vi "Find Run.vi"(0 "Array":dbl[](array[numeric]), 5 "Condition":bool[](array[boolean]), 9 "Midrun index":i32) -> (4 "Run":dbl[](array[numeric]), 6 "Run start index":i32, 8 "Run end index":i32, 10 "Run length":i32)   [LabVIEW 2020]
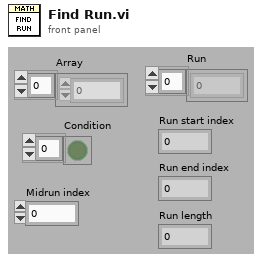
[diagram p1: front panel]
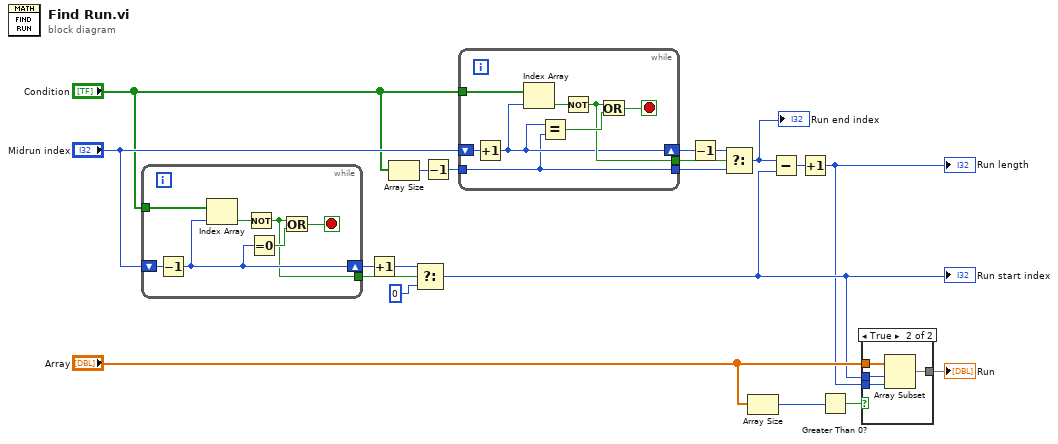
[diagram p0: block diagram]
diagram:
  n1 = while {
    shift-right: [w22] -> w19
    shift-left: "Midrun index" -> [w24]
    tunnel: "Condition" -> [w27]
    tunnel: [w21] -> w20
    stop <- w26 stop-if-true
    n2 = Decrement(x=w24) -> (x-1=w22:i32)
    n3 = Index Array(array=w27, index=w22) -> (element=w25:bool)
    n4 = Not(x=w25) -> (.not. x?=w21:bool)
    n5 = Equal To 0?(x=w22) -> (x = 0?=w23:bool)
    n6 = Or(x=w21, y=w23) -> (x .or. y?=w26:bool)
  }
  n7 = Increment(x=w19) -> (x+1=w18:i32)
  n8 = Array Size(array="Condition") -> (size(s)=w14:i32)
  n9 = Select(t=w18, s=w20, f=0) -> (s? t:f=w2:i32)
  "Run start index" <- w2
  n10 = Decrement(x=w14) -> (x-1=w13:i32)
  n11 = while {
    shift-right: [w29] -> w10
    shift-left: "Midrun index" -> [w32]
    tunnel: "Condition" -> [w35]
    tunnel: [w30] -> w11
    tunnel: w13 -> [w28]
    tunnel: [w28] -> w9
    stop <- w34 stop-if-true
    n12 = Increment(x=w32) -> (x+1=w29:i32)
    n13 = Index Array(array=w35, index=w29) -> (element=w33:bool)
    n14 = Equal?(x=w29, y=w28) -> (x = y?=w31:bool)
    n15 = Not(x=w33) -> (.not. x?=w30:bool)
    n16 = Or(x=w30, y=w31) -> (x .or. y?=w34:bool)
  }
  n17 = Decrement(x=w10) -> (x-1=w12:i32)
  n18 = Select(t=w12, s=w11, f=w9) -> (s? t:f=w8:i32)
  "Run end index" <- w8
  n19 = Array Size(array="Array") -> (size(s)=w3:i32)
  n20 = Subtract(x=w8, y=w2) -> (x-y=w7:i32)
  n21 = Increment(x=w7) -> (x+1=w1:i32)
  "Run length" <- w1
  n22 = Greater Than 0?(x=w3) -> (x > 0?=w4:bool)
  n23 = case shown="True" w4 {
    tunnel: "Array" -> [_ w39]
    tunnel: [_ w38] -> w6
    tunnel: w2 -> [_ w37]
    tunnel: w1 -> [_ w36]
    frame False {
    }
    frame True {
      n24 = Array Subset(array=w39, index=w37, length=w36) -> (w38:dbl[])
    }
  }
  "Run" <- w6
